vi "BatteryDebugColor.vi"() -> ()   [LabVIEW 2019]
uses:
  <vilib>/vision/NI_Vision_Development_Module.lvlib
  sensors.vi
panel:
  out "Color":u32(colorbox)
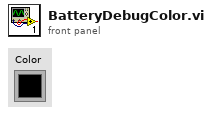
[diagram p1: front panel]
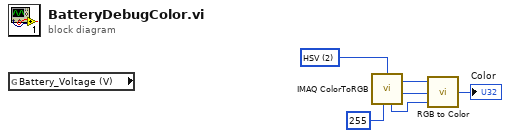
[diagram p0: block diagram]
diagram:
  w6 = u16 2 items=["RGB", "HSL", "HSV", "HSI"] ("Color Mode")
  n1 = global read "sensors.vi" "Battery_Voltage (V)"() -> ()  [unwired: 1 out]
  n2 = call "IMAQ ColorToRGB"("Blue or Luma or Val or Inten value"=u8 255 ("Green or Sat value"), "Color Mode"=w6) -> ("Blue value"=w3:u8, "Green value"=w4:u8, "Red value"=w5:u8)  [unwired: 3 in, 1 out]
  n3 = call <vilib>:"RGB to Color.vi"("B"=w3, "G"=w4, "R"=w5) -> ("Color"=→"Color":u32)
